vi "Global_Telescopio.vi"() -> ()   [LabVIEW 2018]
panel:
  in  "ExecTime":u32
  in  "queueRespCUP":refnum<queue>
  in  "queueCmdCUP":refnum<queue>
  in  "queueRespTUBO":refnum<queue>
  in  "queueCmdTUBO":refnum<queue>
  in  "queueRespDEC":refnum<queue>
  in  "queueCmdDEC":refnum<queue>
  in  "queueRespAH":refnum<queue>
  in  "queueCmdAH":refnum<queue>
  out "PUB AlarmePlataforma":bool
  in  "PUB AtmAlarme":string
  in  "pubDecAcquis":string
  in  "pubRaAcquis":string
  out "versionTCSPD":string="-Versão atual:  01-02-2024;  Versão anterior:   07-06-2023"
  out "dataInAG":string="Panorama"
  in  "BtShutCloseSimul":bool
  out "PUB activeNST":bool
  in  "ExtDEC_shift":string=" 281.52"
  in  "ExtRA_shift":string=" 281.52"
  out "ExtDEC correction":bool
  out "ExtRA correction":bool
  in  "weatherCfgDef":string[](array[string])=["15,000000", "85,000000", "880,000000", "0,000000", "0,000000", "700,000000", "30,000000", "100,000000", "1200,000000", "120,000000"]
  in  "weather160 PUB time":timestamp
  in  "CupTimeLock":u32
  in  "CupLastEnc":string
  in  "RevCupTO":u32
  in  "CupStartPos":i16=2
  in  "QtdEtiquetas":i16=2
  out "PointingModel DEC":dbl
  out "PointingModel RA":dbl
  out "Precessed  DEC":dbl
  out "Precessed RA":dbl
  in  "weather file data":string[](array[string])
  in  "weather file last time":timestamp
  in  "weather 0MQ last time":timestamp
  out "Weather160":T1
  in  "PUB StatShutter":string
  in  "PUB StatDome":string
  in  "PUB PosCup":string
  out "PUB SHUTTER":bool
  out "PUB ObjCentrado":bool
  out "PUB VAR TRACKING":bool
  out "PUB GUIDER":bool
  out "PUB Dome":bool
  out "PUB MOUNT":bool
  out "PUB RA on Target":bool
  out "PUB Mount Fine Movement":bool
  out "PUB Mount Gross Movement":bool
  out "PUB Data Acquisition Activity":bool
  out "PUB Auto guider Activity":bool
  out "PUB Security Zone":bool
  out "PUB Precess Data out-of-date":bool
  out "PUB DEC on Target":bool
  out "PUB Dome on Target":bool
  out "transactionId0MQ":u64
  out "Focuser160":T2
  in  "queuePUSH":refnum<queue>
  in  "queueSUB":refnum<queue>
  in  "Default Met":bool
  in  "Senha LEAF":string
  in  "Flag Leaf":bool
  out "Flag-Rotator":bool
  in  "Hora vent final":string
  in  "Hora vent inicial":string
  in  "Enable ventilador":bool=TRUE
  in  "Caminho camera":string
  in  "DEC AUX":string
  in  "RA AUX":string
  in  "NAME OBJETO AUX":string
  in  "HUM":dbl format="%#_9g"
  in  "BAR":dbl format="%#_9g"
  in  "TEMP":dbl format="%#_9g"
  in  "Habilita supervisao":bool
  in  "Tempo delay":i32=1
  in  "MOTOR LIGADO":string
  in  "Foco":dbl format="%#_9g"
  out "Estado TUBO":i32
  out "Estado DEC":i32
  out "Estado AH":i32
  out "T cup":u32
  out "Estado CUP":i32
  in  "EPOCH AQUIS":string
  in  "Foco Instrumento":string
  in  "Limite EAST":dbl=5.0 min=-12.0 max=12.0 step=0.1
  in  "Limite WEST":dbl=5.0 min=-12.0 max=12.0 step=0.1
  in  "Telescopio":bool
  in  "rotator_def":string=" 281.52"
  out "FinalsFileDownload":bool
  out "Parking":bool
  in  "Tempo Atulização All Sky":i16=1
  in  "Tempo Atulização Cam 3":i16=1
  in  "Tempo Atulização Cam 2":i16=1
  in  "Tempo Atulização Cam 1":i16=1
  in  "Tempo Atulização Cam 0":i16=1
  out "Azimute GRAUS":dbl
  in  "Tabela Proteção":string[][](table)=[["Coude", "281.52", " 11.53", "S", "S", "0.462", "23.1", "23.1"], ["Cassegrain", "281.52", " 11.53", "S", "S", "0.462", "23.1", "23.1"], ["Eucalyptus", "281.52", " 11.53", "S", "S", "0.462", "23.1", "23.1"], ["Cam 1", "281.52", " 11.53", "S", "S", "0.462", "23.1", "23.1"], ["Cam 2", "281.52", " 11.53", "S", "S", "0.462", "23.1", "23.1"], ["Cam IV", "281.52", " 11.53", "S", "S", "0.462", "23.1", "23.1"], ["Polarimetro", "281.52", " 11.53", "S", "S", "0.462", "23.1", "23.1"], ["Fortrap", "281.52", " 11.53", "S", "S", "0.462", "23.1", "23.1"]]
  in  "Raio Máximo":dbl=5.0 min=0.0 max=90.0 step=0.1
  out "AH Zero Local":dbl
  out "DEC Zero Local":dbl
  out "Lista Instrumentos":string[](array[string])
  in  "CalagemDEC_Inicial":string="0.462"
  in  "CalagemAH_Inicial":string="0.462"
  out "CoordDia":bool
  out "AH_now":dbl format="%07.2g"
  in  "Z_LIBERA_GRAUS":dbl
  in  "Z_SEGURANÇA_GRAUS":dbl
  in  "Z_MAX_GRAUS":dbl
  out "LIMITE":bool
  out "STOP ALL":bool
  in  "DestDEC":dbl
  in  "DestCUP":i32
  in  "DestAH":dbl
  out "Bit RX Aquis":bool
  out "Bit RX Guider":bool
  out "AQ Offset Mov":bool
  in  "Air Mass":dbl format="%#_9g"
  out "Correção Aquis":bool
  out "delta_now":dbl format="%07.2g"
  out "aquis_dec":dbl format="%07.2g"
  out "aquis_asc":dbl format="%07.2g"
  out "CorrecaoMin":dbl=0.1
  in  "tel_sts1 Array":bool[](array[boolean])=[TRUE, TRUE, TRUE, TRUE, FALSE, FALSE, TRUE]
  in  "esc_placa":string="0.462"
  in  "guide_esp":string="S"
  in  "guide_cas":string="S"
  in  "guide_ang":string=" 281.52"
  in  "guide_nor":string="  11.53"
  out "Right Ascention":string="00 00 00,00"
  out "Declination":string="00 00 00,00"
  out "Hour Angle":string="00 00 0,00"
  out "Sideral time":string caption="ST"
  out "Zenital angle GRAUS":dbl
  in  "NAME OBJETO":string
  in  "DEC AQUIS":string
  in  "RA AQUIS":string
  out "Centragem Via Aquisicao":bool
  out "AQUISICAO RESOURCE":refnum<visa-resource-name>
  out "Correção Guider":bool
  out "Comunicaçao ok guider":bool
  in  "tel_sts2":u8
  in  "tel_sts1":u8
  out "guide_dec":dbl format="%07.2g"
  out "guide_dir_ns":string
  out "guide_asc":dbl format="%07.2g"
  out "guide_dir_we":string
  out "AUTOGUIDER RESOURCE":refnum<visa-resource-name>
  in  "Data Arq LOG":string="54302.384"
  out "AcumAG DEC":dbl
  out "AcumAG RA":dbl
  out "AcumPrecDEC":dbl
  out "AcumPrecRA":dbl
  out "LatchPrecDEC":dbl
  out "LatchPrecRA":dbl
  out "LatchAG RA":dbl
  out "LatchAG DEC":dbl
  out "CalLocAux DEC":dbl
  out "CalLocAux AH":dbl
  out "CalGlobAux DEC":dbl
  out "CalGlobAux AH":dbl
  in  "ErroMaxCup":i16=2
  out "TargetFOCO":u16
  out "TargetCUP":i16
  out "CalGlobal":bool
  out "CalLocal":bool
  out "ObjCentrado":bool
  out "PosFOCO":u16
  out "PosCUP":i16
  out "PosDEC":dbl
  out "PosAH":dbl
  out "StatusTUBO":bool[](array[boolean])
  out "StatusCUP":bool[](array[boolean])
  out "StatusDEC":bool[](array[boolean])
  out "StatusAH":bool[](array[boolean])
  in  "ErroMaxEixo":dbl=2e-05 format="%.9f"
  out "OffsetCupula":dbl=136.0 format="%#_9g"
  out "CalDEC Local":dbl
  out "CalAH Local":dbl
  out "Calagem DEC":dbl
  out "Calagem AH":dbl
  out "Sideral Time":dbl format="%#_9g"
  out "SYSTEM MESSAGES":string="-Versão atual:  01-02-2024;  Versão anterior:   07-06-2023"
  out "Dome Enable":bool
  in  "Fator Zoom 3":i32
  in  "Fator Zoom 2":i32
  in  "Fator Zoom 1":i32
  in  "Dif DEC":dbl=1.0 format="%.9f"
  in  "Dif RA":dbl=1.0 format="%.9f"
  in  "LimiarRapMed":dbl=0.003 format="%.9f"
  out "TargetRA":dbl
  out "TargetDEC":dbl
  out "Botão GO = STOP":bool
  out "Global Rectangle 3":i32[](array[numeric])
  out "Global Rectangle 2":i32[](array[numeric])
  out "Global Rectangle 1":i32[](array[numeric])
  out "P2":i32[](array[numeric])
  out "P1":i32[](array[numeric])
  out "P0":i32[](array[numeric])
  in  "HORIZONTAL":i32(slide) scale=0.0..400.0
  in  "VERTICAL":i32(slide)
  out "Nome Image Aux 3":string="Panorama"
  out "Nome Image Cam 3":string="Panorama"
  out "Nome Image Aux 2":string="Panorama"
  out "Nome Image Aux":string="Panorama"
  out "Nome Image Cam 2":string="Panorama"
  out "Nome Image Cam1":string="Panorama"
  in  "OffsetZ":dbl format="%#_11g"
  in  "OffsetY":dbl format="%#_11g"
  in  "OffsetX":dbl format="%#_11g"
  in  "DistEixos":dbl format="%#_11g"
  in  "RaioCup":dbl format="%#_11g"
  in  "LATrad":dbl format="%#_11g"
  out "ativar botão SET":bool
  out "ativar botão GO":bool
  out "working area = VERDE":bool
  out "desativar botão GO":bool
  out "Piscar working area":bool
  in  "Caminho Estação Meteorológica":string="\\\\200.131.64.185\\clima\\download.txt"
  in  "Erro Canal 4":bool
  in  "Erro Canal 3":bool
  in  "Erro Canal 2":bool
  in  "Erro Canal 1":bool
  out "String  Recebido Canal 4":string
  out "String  Recebido Canal 3":string
  out "String  Recebido Canal 2":string
  out "String  Recebido Canal 1":string
  in  "HABILITA ENV. Canal 4":bool
  out "String Enviado Canal 4":string
  in  "HABILITA ENV. Canal 3":bool
  out "String Enviado Canal 3":string
  in  "HABILITA ENV. Canal 2":bool
  out "String Enviado Canal 2":string
  in  "HABILITA ENV. Canal 1":bool
  out "String Enviado Canal 1":string
  out "Temperatura":dbl
  out "URL Temperatura":string
  out "Instrum":u16
  out "Controller Rem/Loc":i32
  out "Dados do Computador Remoto Conectado":T3(array[cluster])
  in  "Habilita Servidor":bool
  in  "stop":bool
  # "Datasocket"
  # "V 1.0.21: Obsoleto. Usado 0MQ."
  # "*"
  # "*"
  # "Horas"
  # "Horas"
  # "Graus"
  # "Autoguider"
  # "*"
  # "arcsec"
  # "arcsec"
  # "*"
  # "MUDANÇA 08/04/2011:\nFoi deletada uma caixa de texto (label = \"SYSTEM MESSAGES\", mesmo nome de outra global) que não estava sendo usada."
  # "AQUISI敲O VIA COMPUTADOR LINUX"
  # "Armazena ckeck-box \"Default Met\" da aba\nEstação Meteor. de Configuração.vi"
  # "ZeroMQ"
  # "TCSPD Status PUB"
  # "PUB FOCUSER160\n{\n\"absolute\": true,\n\"alarm\": false,\n\"broker\": \"Focuser160\",\n\"cmd\": {\n    \"clientId\": 1234,\n    \"clientTransactionId\": 9876,\n     \"clientName\": \"TCSPD\",\n     \"action\": {\"move\" : 10\"}\n     },\n\"connected\": true,\n\"controller\": \"Focuser160\",\n\"device\": \"Mirror2\",\n\"error\": \"\",\n\"homing\": false,\n\"initialized\": true,\n\"isMoving\": false,\n\"maxSpeed\": 150,\n\"maxStep\": 1000000,\n\"position\": 1549,\n\"tempComp\": false,\n\"tempCompAvailable\": false,\n“temperature”: 22,\n\"timestamp\": \"2000-10-31T01:30:00.123\",\n\"version\": \"1.0.0\"\n}"
  # "Faixa do Azimute\n   De:              Ate:"
  # "Ângulo Zenital\n  Máx:       Segur.:       Libera:"
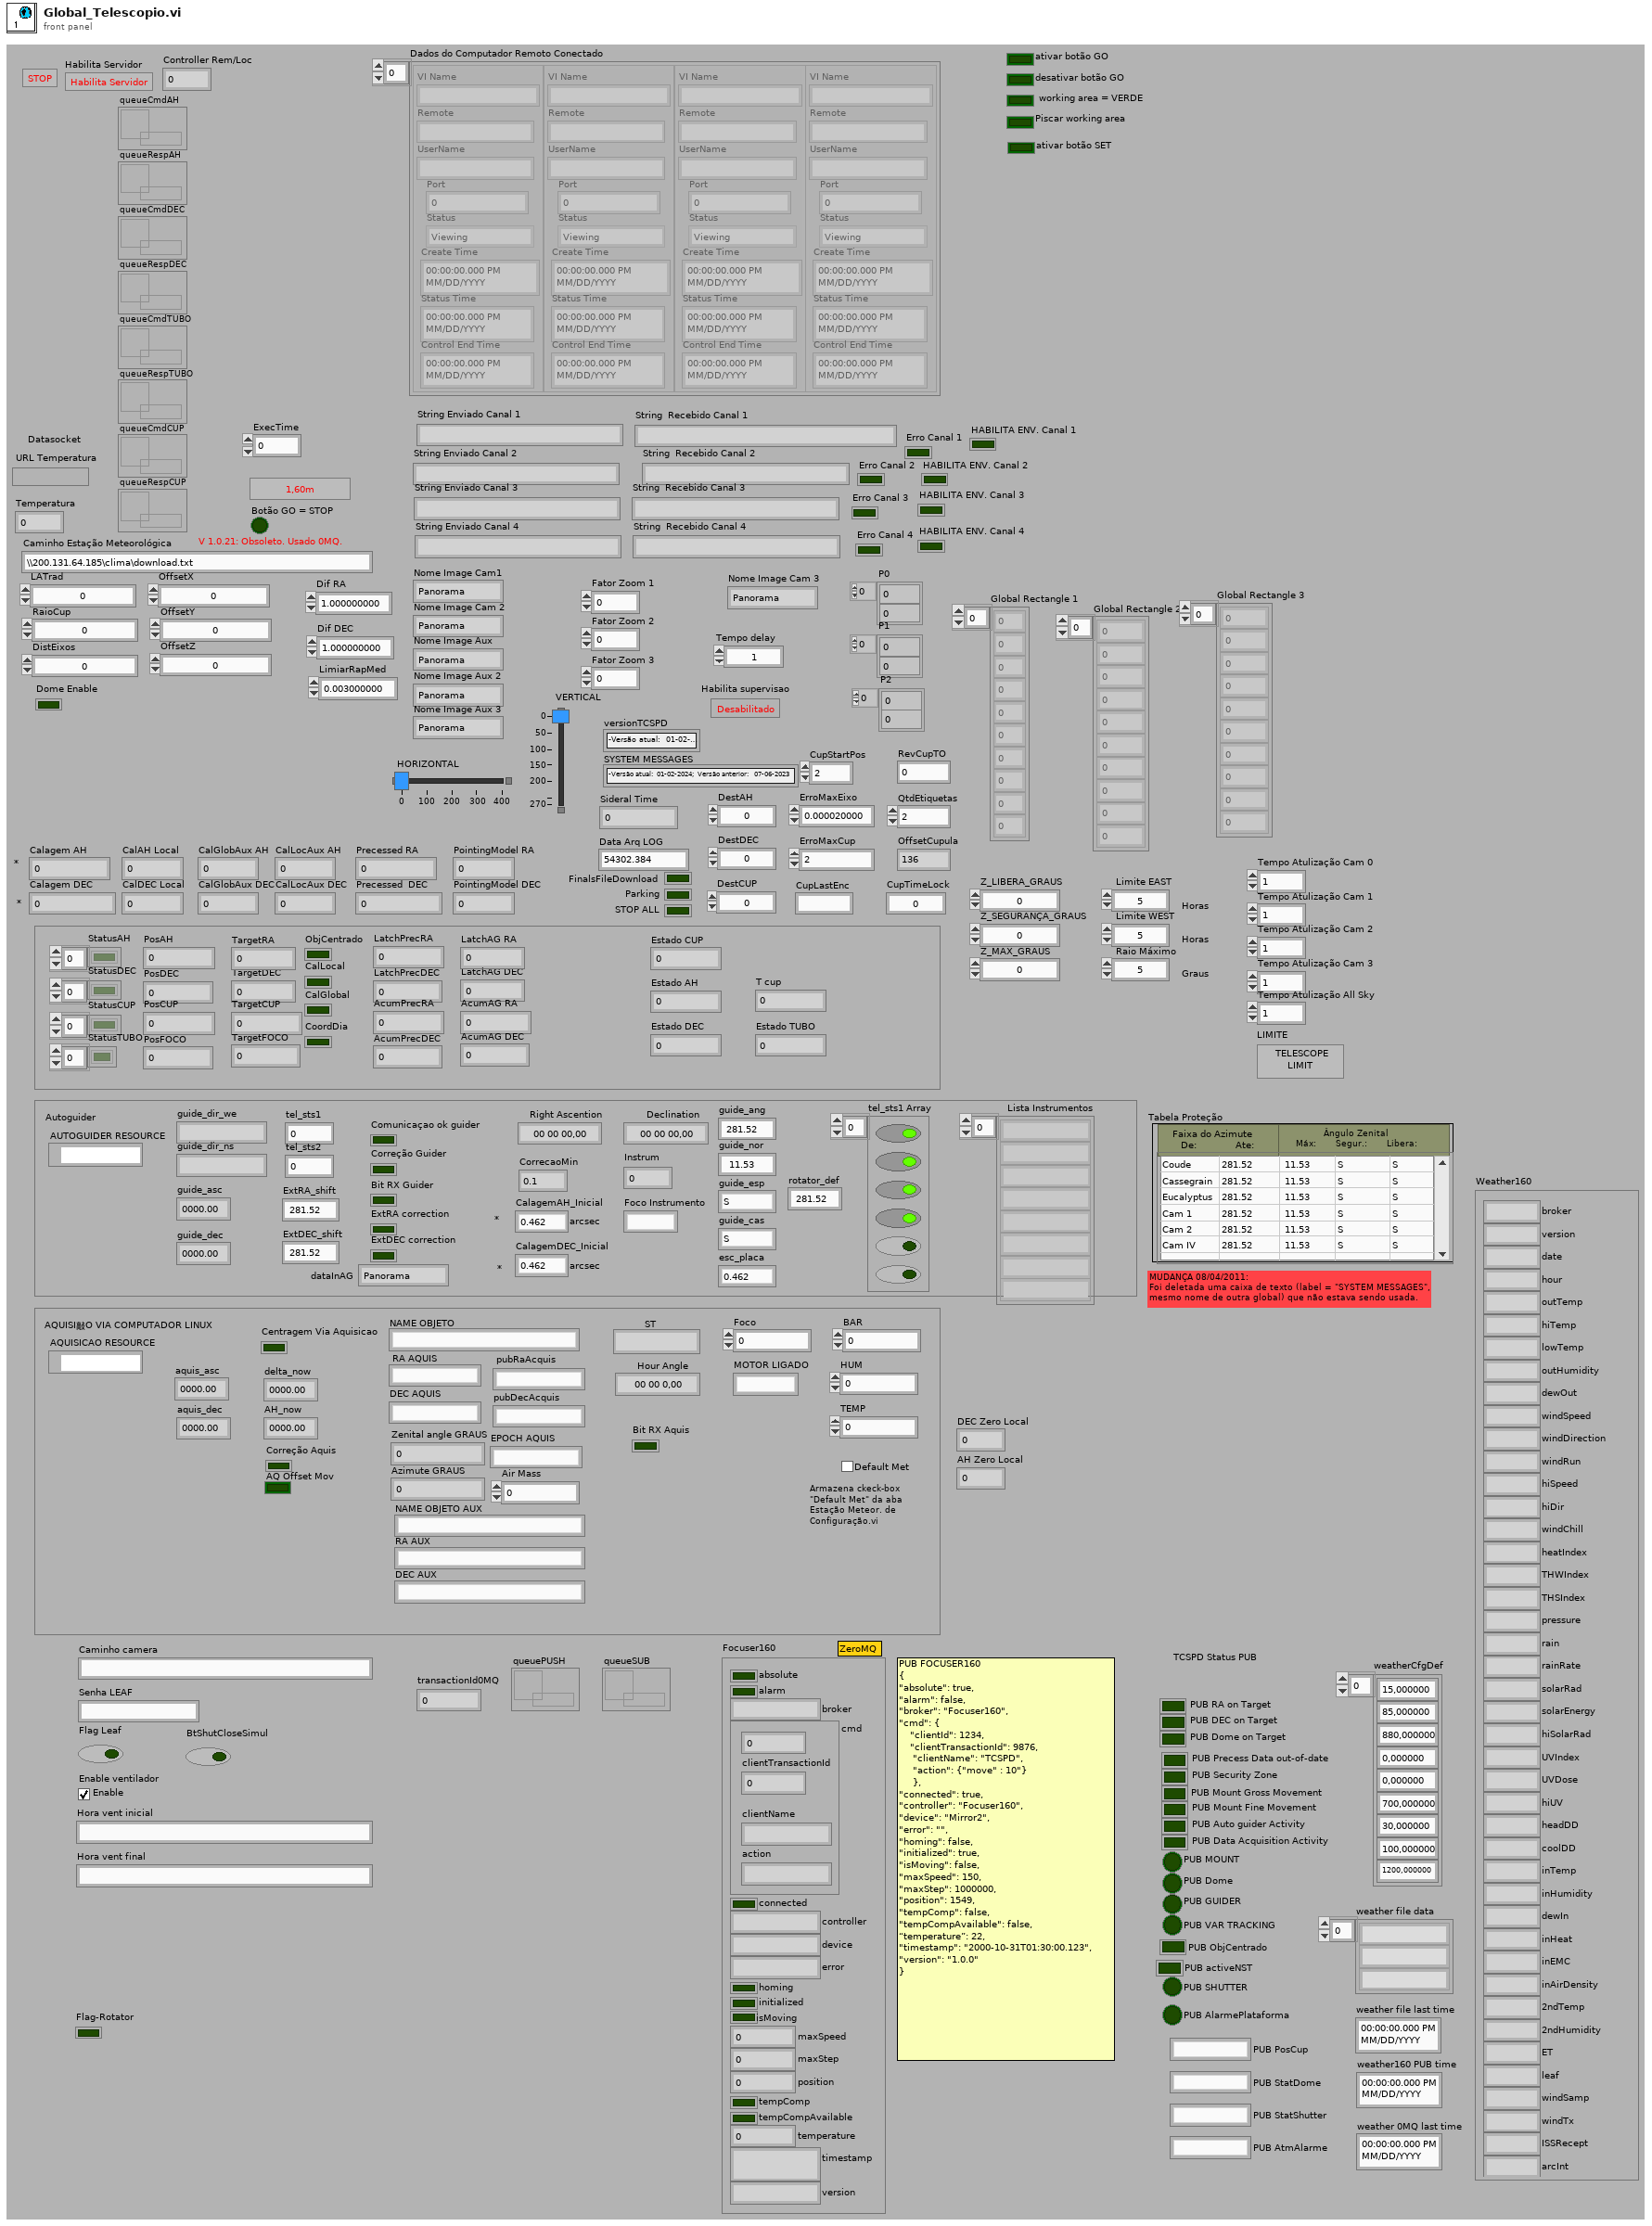
[diagram p1: front panel]
types:
  T1 = cluster{"broker":string, "version":string, "date":string, "hour":string, "outTemp":string, "hiTemp":string, "lowTemp":string, "outHumidity":string, "dewOut":string, "windSpeed":string, "windDirection":string, "windRun":string, "hiSpeed":string, "hiDir":string, "windChill":string, "heatIndex":string, "THWIndex":string, "THSIndex":string, "pressure":string, "rain":string, "rainRate":string, "solarRad":string, "solarEnergy":string, "hiSolarRad":string, "UVIndex":string, "UVDose":string, "hiUV":string, "headDD":string, "coolDD":string, "inTemp":string, "inHumidity":string, "inHeat":string, "inEMC":string, "inAirDensity":string, "2ndTemp":string, "2ndHumidity":string, "ET":string, "leaf":string, "windSamp":string, "windTx":string, "ISSRecept":string, "dewIn":string, "arcInt":string}
  T2 = cluster{"absolute":bool, "alarm":bool, "broker":string, "cmd":cluster{"clientId":dbl, "clientTransactionId":dbl, "clientName":string, "action":string}, "connected":bool, "controller":string, "device":string, "error":string, "homing":bool, "initialized":bool, "isMoving":bool, "maxSpeed":dbl, "maxStep":dbl, "position":dbl, "tempComp":bool, "tempCompAvailable":bool, "temperature":dbl, "timestamp":string, "version":string}
  T3 = cluster{"VI Name":string, "Remote":string, "UserName":string, "Port":i32, "Status":enum32{"Viewing", "Waiting For Control", "Controlling"}, "Create Time":timestamp, "Status Time":timestamp, "Control End Time":timestamp}[]
diagram:
